vi "ExSubGetTemp.vi"(0 "Camera Handle":u32, 1 "error in (no error)":errorcluster) -> (2 "Camera Handle":u32, 3 "Temperature Real":dbl format="%.2f", 4 "error out":errorcluster)   [LabVIEW 2010]
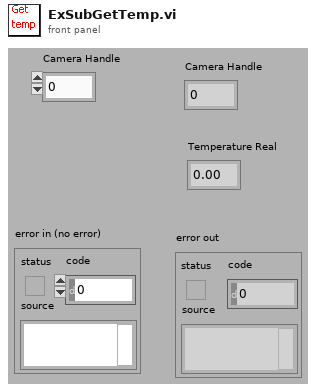
[diagram p1: front panel]
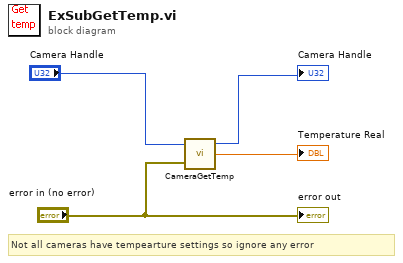
[diagram p0: block diagram]
diagram:
  # "Not all cameras have tempearture settings so ignore any error"
  n1 = call <userlib>:"CameraGetTemp.vi"("Camera Handle"="Camera Handle", "error in (no error)"="error in (no error)") -> ("Camera Handle"=→"Camera Handle":u32, "Temperature"=→"Temperature Real":dbl)  [unwired: 1 out]
  "error out" <- "error in (no error)"
